vi "UIRef.vi"(8 "error in":errorcluster, 11 "Tagbus PID Module editor node in":refnum<class "Tagbus PID Module editor node.lvclass">) -> (0 "error out":errorcluster, 2 "VI refnum":refnum<vi>, 3 "Tagbus PID Module editor node out":refnum<class "Tagbus PID Module editor node.lvclass">)   [LabVIEW 2014, in "Tagbus PID Module editor node.lvclass"]
uses:
  Tagbus PID Module editor node.lvclass
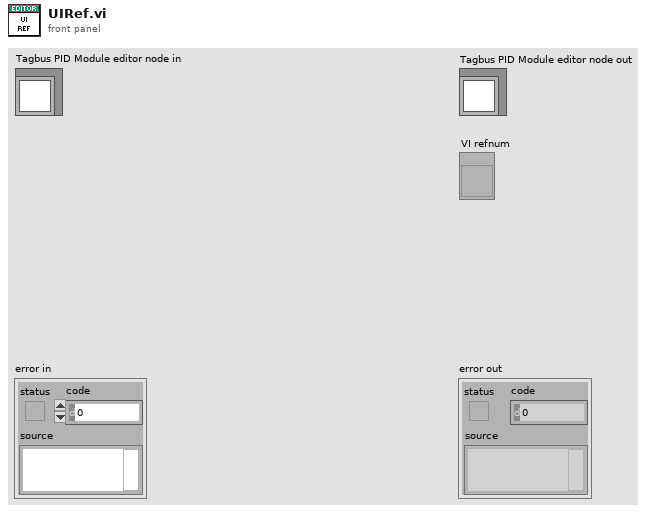
[diagram p1: front panel]
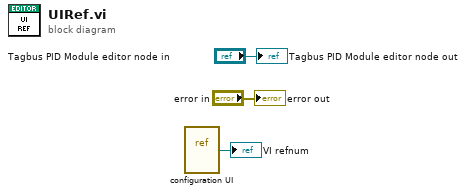
[diagram p0: block diagram]
diagram:
  n1 = vi-ref "configuration UI.vi"() -> (→"VI refnum":refnum<vi>)
  "error out" <- "error in"
  "Tagbus PID Module editor node out" <- "Tagbus PID Module editor node in"
